vi "forceSetpoint.vi"(8 "error in (no error)":errorcluster, 10 "Force Demand":T1 min=-888.0 max=888.0 format="%.2f", 11 "Context in":refnum<class "Context.lvclass">) -> (0 "error out":errorcluster, 3 "Context out":refnum<class "Context.lvclass">)   [LabVIEW 2013, in "Context.lvclass"]
uses:
  Context.lvclass
  Typedefs/ForceDemand.ctl
  Context.lvclass/Context.ctl
  State/State.lvclass
  Model/Model/Model.lvclass
  Typedefs/FAMTTypedefs.lvlib
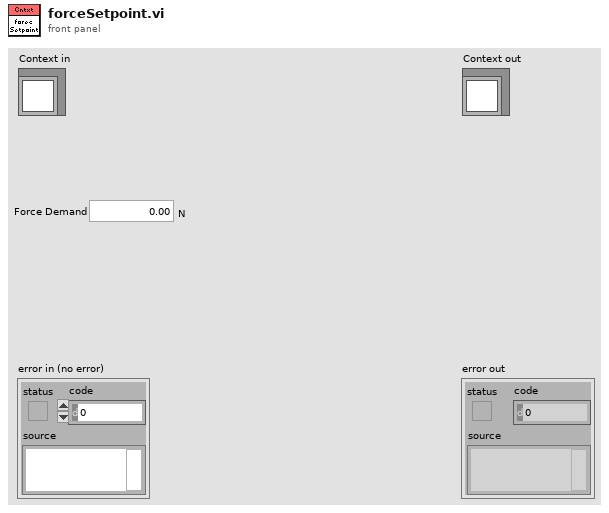
[diagram p1: front panel]
types:
  T1 = typedef "FAMTTypedefs.lvlib/ForceDemand.ctl" = dbl[unit]
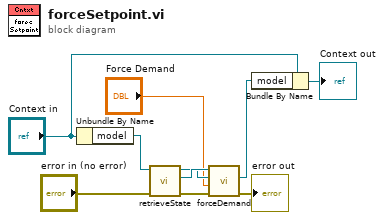
[diagram p0: block diagram]
diagram:
  n1 = Unbundle By Name("Context in") -> ("model"=w9:refnum<class "Model.lvclass">)
  n2 = call "retrieveState.vi"("error in (no error)"="error in (no error)", "Model in"=w9) -> ("error out"=w2:errorcluster, "state"=w10:refnum<class "State.lvclass">, "Model out"=w8:refnum<class "Model.lvclass">)  [unwired: 7 in]
  n3 = call-dynamic "forceDemand.vi"("error in (no error)"=w2, "Force Demand"="Force Demand", "model"=w8, "State in"=w10) -> ("error out"=→"error out":errorcluster, "model 2"=w5:refnum<class "Model.lvclass">)  [unwired: 5 in, 1 out]
  n4 = Bundle By Name(cluster="Context in", "model"=w5) -> (→"Context out":refnum<class "Context.lvclass">)
